vi "libdaq_adc_send_trigger.vi"(0 "error in (no error)":errorcluster, 1 "device_name":string, 2 "module_name":string) -> (14 "error out":errorcluster, 15 "device_name":string, 16 "module_name":string)   [LabVIEW 2022 SP3, in "libdaqVI.lvlib"]
doc: "发送ADC软件采样触发信号，DAQ设备收到触发信号后ADC开始采样"
uses:
  libdaqVI.lvlib
  dll/daqlib.dll
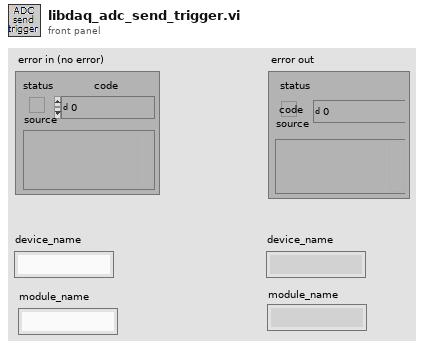
[diagram p1: front panel]
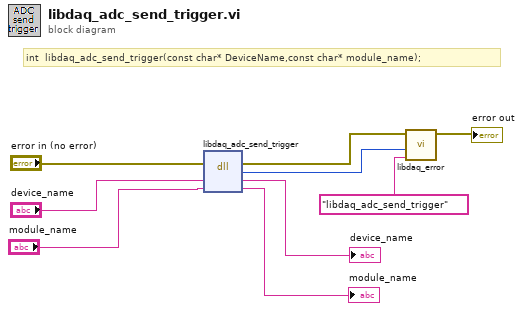
[diagram p0: block diagram]
diagram:
  # "int  libdaq_adc_send_trigger(const char* DeviceName,const char* module_name);"
  n1 = dll-call lib="D:/Labview_projects/DAQ_USB3212/libdaqVI/dll/daqlib.dll" fn="libdaq_adc_send_trigger"(error in="error in (no error)", "device_name"="device_name", "module_name"="module_name") -> (error out=w3:errorcluster, "return type"=w2:i32, "device_name"=→"device_name":string, "module_name"=→"module_name":string)  [unwired: 2 in, 1 out]
  n2 = call "libdaq_error.vi"("error source"="libdaq_adc_send_trigger", "error code"=w2, "错误输入（无错误）"=w3) -> ("错误输出"=→"error out":errorcluster)  [unwired: 8 in]
